vi "DO Write Port.vi"(8 "error in (no error)":errorcluster caption="错误输入（无错误）", 9 "Value":u32, 10 "Port":u16, 11 "CardNumber":u16) -> (0 "error out":errorcluster caption="错误输出", 3 "function return":i16)   [LabVIEW 2017, in "Adlink IO.lvlib"]
doc: "I16 __stdcall DO_WritePort(U16 CardNumber, U16 Port, U32 Value);"
uses:
  Adlink IO.lvlib
  PCI-Dask.dll
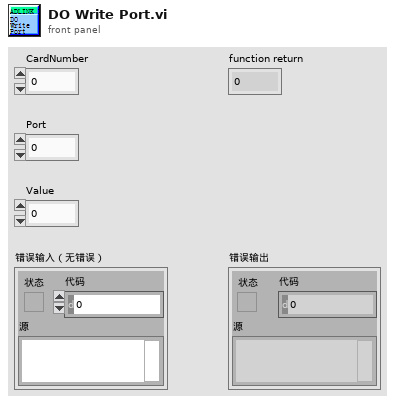
[diagram p1: front panel]
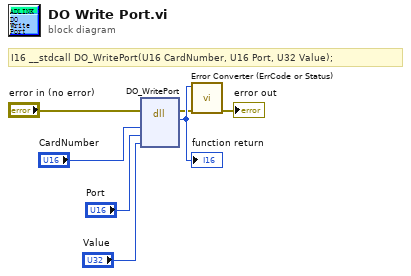
[diagram p0: block diagram]
diagram:
  # "I16 __stdcall DO_WritePort(U16 CardNumber, U16 Port, U32 Value);"
  n1 = dll-call lib="PTH2Jabs E迈治LV范例testSubVIsADLINKIO\tAdlink IO\nPCI-Dask.*" fn="DO_WritePort"(error in="error in (no error)", "CardNumber"="CardNumber", "Port"="Port", "Value"="Value") -> (error out=w2:errorcluster, w7:i16)  [unwired: 5 in, 1 out]
  "function return" <- w7
  n2 = call "Error Converter (ErrCode or Status).vi"("error in (no error)"=w2, "error code"=w7) -> ("error out"=→"error out":errorcluster)  [unwired: 9 in]
